vi "Generate New Name.vi"(8 "error in (no error)":errorcluster, 10 "Default Name":string="New Step", 11 "Project in":refnum<class "Project.lvclass">) -> (0 "error out":errorcluster, 2 "Name":string, 3 "Project out":refnum<class "Project.lvclass">)   [LabVIEW 2015, in "Editor.lvclass"]
uses:
  Editor.lvclass
  Project.lvclass
  Step.lvclass
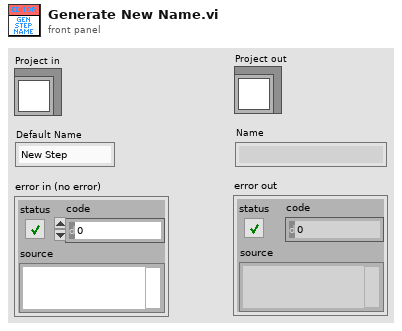
[diagram p1: front panel]
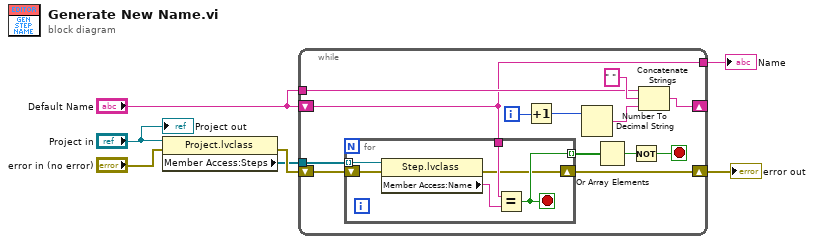
[diagram p0: block diagram]
diagram:
  n1 = property class="Project.lvclass"(reference="Project in", error in="error in (no error)") -> (error out=w5:errorcluster, "Member Access:Steps"=w4:refnum<class "Step.lvclass">[])  [unwired: 1 out]
  n2 = while {
    tunnel: w4 -> [w20]
    shift-right: [w13] -> _
    shift-left: "Default Name" -> [w8]
    tunnel: "Default Name" -> [w9]
    shift-right: [w10] -> w2
    shift-left: w5 -> [w19]
    tunnel: [w8] -> w1
    i -> [w16]
    stop <- w11 stop-if-true
    n3 = for {
      tunnel: w20 -> [w26] mode=indexing
      tunnel: w8 -> [w23]
      tunnel: [w22] -> w18 mode=indexing
      shift-right: [w21] -> w10
      shift-left: w19 -> [w25]
      stop <- w22 stop-if-true
      n4 = property class="Step.lvclass"(reference=w26, error in=w25) -> (error out=w21:errorcluster, "Member Access:Name"=w24:string)  [unwired: 1 out]
      n5 = Equal?(x=w23, y=w24) -> (x = y?=w22:bool)
    }
    n6 = Increment(x=w16) -> (x+1=w15:i32)
    n7 = Number To Decimal String(number=w15) -> (decimal integer string=w14:string)  [unwired: 1 in]
    n8 = Or Array Elements(Boolean array=w18) -> (logical OR=w12:bool)
    n9 = Not(x=w12) -> (.not. x?=w11:bool)
    n10 = Concatenate Strings(w9, " ", w14) -> (w13:string)
  }
  "error out" <- w2
  "Name" <- w1
  "Project out" <- "Project in"
